vi "tictoc_FGV.vi"(7 "Error In":errorcluster, 10 "Case":enum16{"tic", "toc"}(ring)) -> (0 "Error Out":errorcluster, 2 "Elapsed Time (s)":dbl)   [LabVIEW 2017]
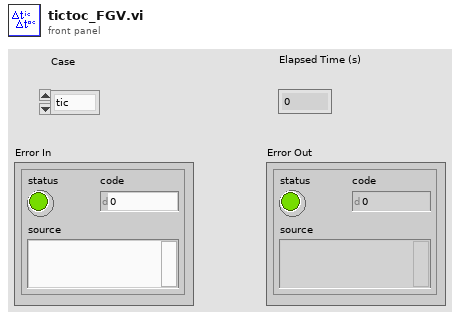
[diagram p1: front panel]
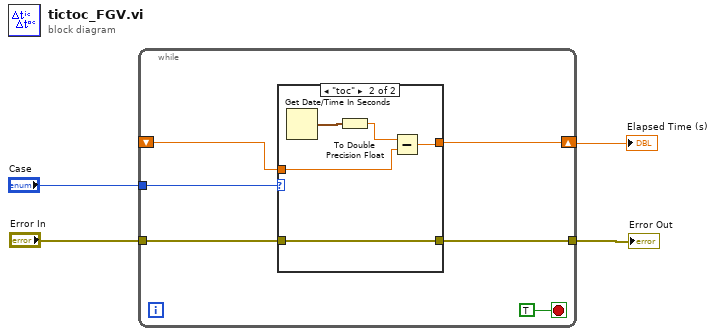
[diagram p0: block diagram]
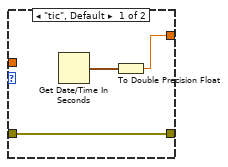
[diagram p2: hidden frame]
diagram:
  n1 = while {
    tunnel: "Case" -> [w10]
    shift-right: [w6] -> w1
    shift-left: _ -> [w7]
    tunnel: "Error In" -> [w9]
    tunnel: [w8] -> w2
    stop <- TRUE stop-if-true
    n2 = case shown="\"toc\"" w10 {
      tunnel: w9 -> [w13 w18]
      tunnel: [w13 w18] -> w8
      tunnel: w7 -> [_ w16]
      tunnel: [w11 w14] -> w6
      frame "tic", Default {
        n3 = Get Date/Time In Seconds() -> (seconds since 1Jan1904=w12:timestamp)
        n4 = To Double Precision Float(number=w12) -> (double precision float=w11:dbl)
      }
      frame "toc" {
        n5 = Get Date/Time In Seconds() -> (seconds since 1Jan1904=w17:timestamp)
        n6 = To Double Precision Float(number=w17) -> (double precision float=w15:dbl)
        n7 = Subtract(x=w15, y=w16) -> (x-y=w14:dbl)
      }
    }
  }
  "Error Out" <- w2
  "Elapsed Time (s)" <- w1
